vi "ShowWaitTime.vi"(1 "Delay (sec)":dbl format="%.2f") -> (0 "GS200 program \nis  running\nWAIT (sec)":dbl format="%.2f")   [LabVIEW 2020]
doc: "NOTE: This VI was built to be used in conjunction with either Automatic VI Server Connection Polling.vi or Manual VI Server Connection Polling.vi. For instructions, see either of these VI Server Connection Polling VIs. When run, this VI will keep track of its elapsed time."
uses:
  Instance           2 43Saved   VI Server Connection Polling Target .vi
  Instance           1 43Saved   VI Server Connection Polling Target .vi
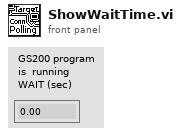
[diagram p1: front panel]
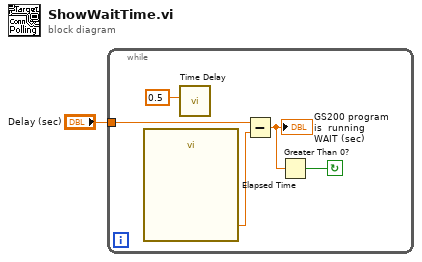
[diagram p0: block diagram]
diagram:
  n1 = while {
    tunnel: "Delay (sec)" -> [w4]
    stop <- w2 continue-if-true
    n2 = call "Elapsed Time"() -> ("Elapsed Time (s)"=w5:dbl)  [unwired: 12 in, 7 out]
    n3 = call "Time Delay"("Delay Time (s)"=0.5) -> ()  [unwired: 10 in, 1 out]
    n4 = Subtract(x=w4, y=w5) -> (x-y=w3:dbl)
    "GS200 program \nis  running\nWAIT (sec)" <- w3
    n5 = Greater Than 0?(x=w3) -> (x > 0?=w2:bool)
  }
